vi "DVR Q Top Level.vi"() -> ()   [LabVIEW 2021, in "DVR Qs.lvlib"]
uses:
  DVR Qs.lvlib
panel:
  in  "Numeric Control":i32
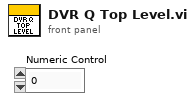
[diagram p1: front panel]
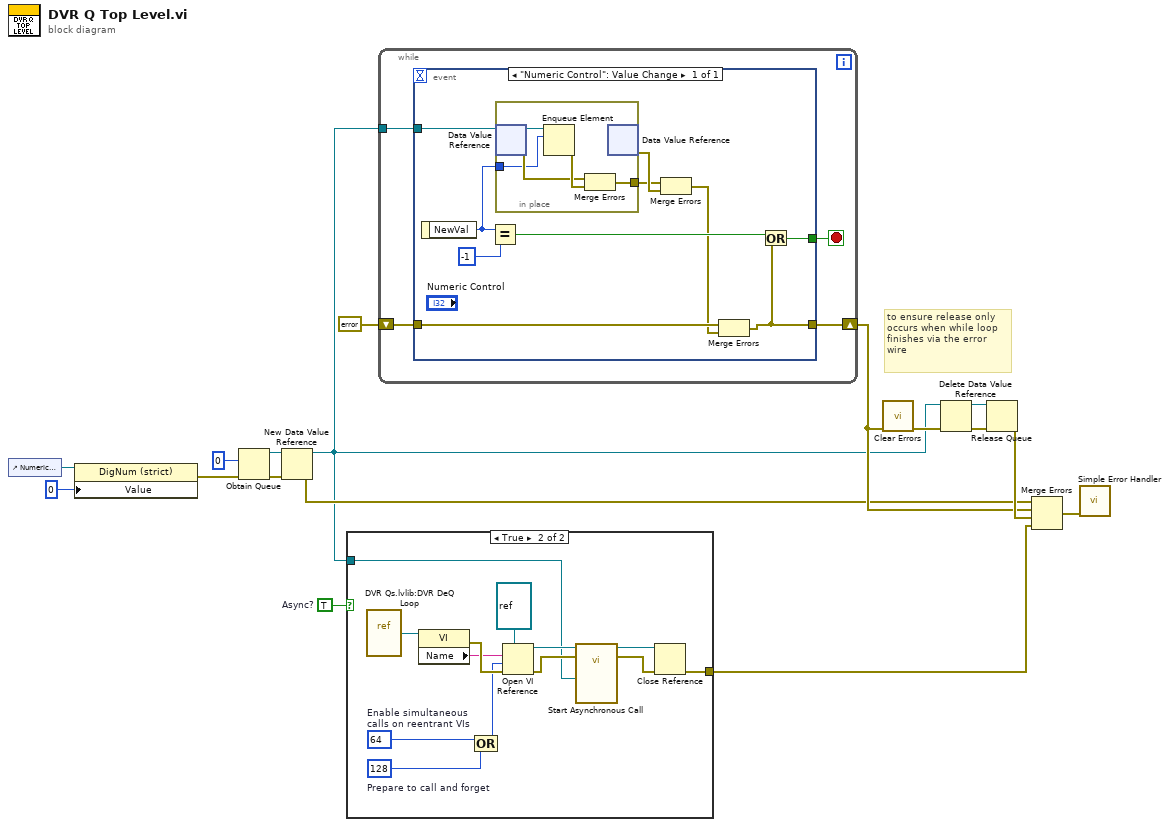
[diagram p0: block diagram]
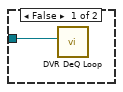
[diagram p2: hidden frame]
diagram:
  w9 = TRUE  # Async?
  # "to ensure release only occurs when while loop finishes via the error wire"
  n1 = control-ref of="Numeric Control"() -> (w17:refnum<vi>)
  n2 = property class="DigNum (strict)"(reference=w17, "Value"=0) -> (error out=w13:errorcluster)  [unwired: 1 in, 1 out]
  n3 = Obtain Queue(element data type=0 ("I32"), error in (no error)=w13) -> (queue out=w4:refnum<queue>, error out=w3:errorcluster)  [unwired: 3 in, 1 out]
  n4 = New Data Value Reference(data value=w4, error in=w3) -> (data value reference=w1:refnum<data-value>, error out=w2:errorcluster)
  n5 = case shown="True" w9 {
    tunnel: w1 -> [w18 w19]
    tunnel: [_ w20] -> w8
    frame False {
      n6 = call "DVR DeQ Loop.vi"("DVR Q"=w18) -> ()  [unwired: 11 in]
    }
    frame True {
      w26 = 128  # Prepare to call and forget
      w27 = 64  # Enable simultaneous calls on reentrant VIs
      n7 = vi-ref "DVR Qs.lvlib:DVR DeQ Loop.vi"() -> (w30:refnum<vi>)
      n8 = property class="VI"(reference=w30) -> (error out=w29:errorcluster, "Name"=w28:string)  [unwired: 1 in, 1 out]
      n9 = Compound Arithmetic op=OR(w27, w26) -> (w25:i32)
      n10 = Open VI Reference(type specifier VI Refnum (for type only)=refnum<vi> refnum, vi path=w28, options=w25, error in (no error)=w29) -> (vi reference=w23:refnum<vi>, error out=w24:errorcluster)  [unwired: 2 in]
      n11 = call-by-ref "Start Asynchronous Call"(reference=w23, error in=w24, "DVR Q"=w19) -> (reference out=w21:refnum<vi>, error out=w22:errorcluster)  [unwired: 11 in]
      n12 = Close Reference(reference=w21, error in (no error)=w22) -> (error out=w20:errorcluster)
    }
  }
  n13 = while {
    shift-right: [w34] -> w10
    shift-left: errorcluster {"status"=FALSE, "code"=0, "source"=""} ("error IO") -> [w33]
    tunnel: w1 -> [w32]
    stop <- w35 stop-if-true
    n14 = event shown="[0] \"Numeric Control\": Value Change" {
      selector: _ -> [_]
      dyn-events: _ -> [_]
      timeout: _ -> [_]
      tunnel: w32 -> [w40]
      tunnel: [w42] -> w35
      tunnel: [w41] -> w34
      tunnel: w33 -> [w43]
      event "Numeric Control": Value Change {
        n15 = event-data() -> ("NewVal"=w39:i32)  [unwired: 1 in]
        n16 = Equal?(x=w39, y=-1) -> (x = y?=w44:bool)
        n17 = in-place {
          in-place-border: [w48] -> w37
          in-place-border: w39 -> [w46]
          n18 = in-place-dvr #1(w40) -> (w50:refnum<queue>, w47:errorcluster)
          n19 = Enqueue Element(queue=w50, element=w46) -> (error out=w49:errorcluster)  [unwired: 2 in, 2 out]
          n20 = Merge Errors(w47, w49) -> (w48:errorcluster)
          n21 = in-place-dvr #1() -> (w38:errorcluster)  [unwired: 1 in, 1 out]
        }
        n22 = Merge Errors(w37, w38) -> (w36:errorcluster)
        n23 = Merge Errors(w43, w36) -> (w41:errorcluster)
        n24 = Or(x=w44, y=w41) -> (x .or. y?=w42:bool)
      }
    }
  }
  n25 = call <vilib>:"Clear Errors.vi"("error in (no error)"=w10) -> ("error out"=w6:errorcluster)  [unwired: 5 in, 1 out]
  n26 = Delete Data Value Reference(data value reference=w1, error in=w6) -> (data value=w7:refnum<queue>, error out=w5:errorcluster)
  n27 = Release Queue(queue=w7, error in (no error)=w5) -> (error out=w11:errorcluster)  [unwired: 1 in, 2 out]
  n28 = Merge Errors(w2, w10, w11, w8) -> (w14:errorcluster)
  n29 = call <vilib>:"Simple Error Handler.vi"("error in (no error)"=w14) -> ()  [unwired: 4 in, 5 out]
